vi "3.3-Get Ground Magnitude.vi"() -> (0 "Numeric":dbl)   [LabVIEW 2010]
uses:
  3.0-Global.vi
panel:
  out "Lidar Degree":dbl
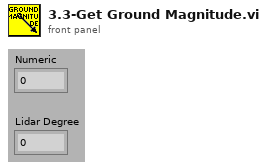
[diagram p1: front panel]
types:
  T1 = typedef "2.1 Act Debug.ctl" = cluster{"Drive":cluster{"2.1 Drive Control Voltage":fxp<+/-,20,5>, "2.1 Drive PID Output":fxp<+/-,20,5>, "2.1.1 Drive Error":fxp<+/-,18,1>, "2.1.1 Drive Error I":fxp<+/-,64,46>, "2.1.1 Drive Error D":fxp<+/-,18,1>, "Motor Speed Integer":fxp<+/-,10,8>, "Drive Position Integer":i32}, "Steering":cluster{"2.1  Steering Control Voltage":fxp<+/-,20,5>, "2.1  Steering Lead Output":fxp<+/-,20,5>, "Steering V":fxp<+/-,10,8>, "Steering Position Integer":i32, "2.1.2 sqrt(10)s+bdt":fxp<+/-,18,20>, "2.1.2 (sqrt(10)s+bdt)/(s/sqrt(10)+bdt)":fxp<+/-,20,22>, "2.1.2 s(sqrt(10)s+bdt)/(s/sqrt(10)+bdt)":fxp<+/-,20,22>}, "Lidar":cluster{"2.1  Lidar Control Voltage":fxp<+/-,20,5>, "2.1  Lidar PID Output":fxp<+/-,20,5>, "2.1.3 Lidar Error":fxp<+/-,18,1>, "2.1.3 Lidar Error I":fxp<+/-,64,46>, "2.1.3 Lidar Error D":fxp<+/-,18,1>, "Lidar Position Integer":i32, "Lidar Motor Position Integer":i32}}
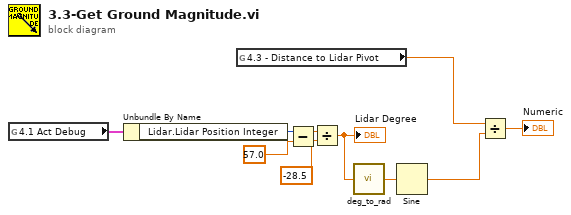
[diagram p0: block diagram]
diagram:
  n1 = global read "3.0-Global.vi" "4.1 Act Debug"() -> (w3:T1)
  n2 = Unbundle By Name(w3) -> ("Lidar.Lidar Position Integer"=w1:i32)
  n3 = global read "3.0-Global.vi" "4.3 - Distance to Lidar Pivot"() -> (w8:dbl)
  n4 = Subtract(x=w1, y=57.0 ("Lidar Offset")) -> (x-y=w4:dbl)
  n5 = Divide(x=w4, y=-28.5 ("Lidar Scale")) -> (x/y=w6:dbl)
  "Lidar Degree" <- w6
  n6 = call "deg_to_rad.vi"("Degrees"=w6) -> ("Radians"=w7:dbl)
  n7 = Sine(x=w7) -> (sin(x)=w9:dbl)
  n8 = Divide(x=w8, y=w9) -> (x/y=→"Numeric":dbl)
